vi "Correggi separatore decimale.vi"(10 "Array in":string[][](array[string])) -> (3 "Array out":string[][](array[string]))   [LabVIEW 2019]
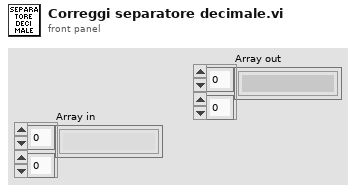
[diagram p1: front panel]
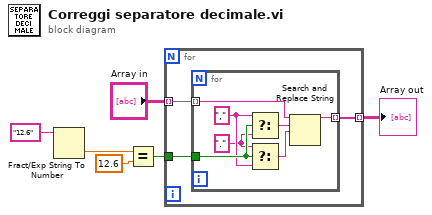
[diagram p0: block diagram]
diagram:
  n1 = Fract/Exp String To Number(string="12.6") -> (number=w3:dbl)  [unwired: 3 in, 1 out]
  n2 = Equal?(x=w3, y=12.6) -> (x = y?=w1:bool)
  n3 = for {
    tunnel: "Array in" -> [w9] mode=indexing
    tunnel: w1 -> [w8]
    tunnel: [w7] -> w6 mode=indexing
    n4 = for {
      tunnel: w9 -> [w16] mode=indexing
      tunnel: w8 -> [w14]
      tunnel: [w10] -> w7 mode=indexing
      w11 = "."
      w12 = ","
      n5 = Select(t=w12, s=w14, f=w11) -> (s? t:f=w15:string)
      n6 = Select(t=w11, s=w14, f=w12) -> (s? t:f=w13:string)
      n7 = Search and Replace String(input string=w16, search string=w15, replace string=w13) -> (result string=w10:string)  [unwired: 5 in, 3 out]
    }
  }
  "Array out" <- w6
